vi "proptest_instancecount.vi"() -> (0 "err 538301":errorcluster, 2 "no support=ok":bool)   [LabVIEW 2025, in "NISE_CEF_Tests.lvlib"]
uses:
  NISE_CEF_Tests.lvlib
  Trunk/Configuration Framework/serializable configuration/NISE_CEF_serializable configuration.lvclass
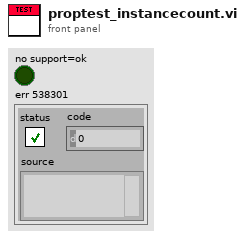
[diagram p1: front panel]
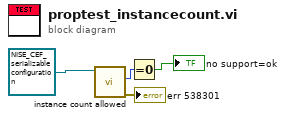
[diagram p0: block diagram]
diagram:
  n1 = call-dynamic "instance count allowed.vi"("configuration in"=refnum<class "NISE_CEF_serializable configuration.lvclass"> refnum ("configuration")) -> ("error out"=→"err 538301":errorcluster, "instances allowed"=w3:i32)  [unwired: 8 in, 1 out]
  n2 = Equal To 0?(x=w3) -> (x = 0?=→"no support=ok":bool)
